vi "Movement sample.vi"() -> ()   [LabVIEW 2018]
uses:
  Underlying VI's/Motor Control VI with PID/MOTOR CONTROL WITH PID AE DIRECTION TYPE DEF.ctl
  Underlying VI's/NavX VI/navX type def.ctl
  Underlying VI's/Motor Control VI with PID/MOTOR CONTROL WITH PID AE DATA MODE TYPE DEF.ctl
  <vilib>/Studica/Studica Toolkit/Background/I2C Channel.ctl
  <vilib>/Studica/Studica Toolkit/NavX/NavX.lvlib
  <vilib>/Studica/Studica Toolkit/Background/DIO Channel.ctl
panel:
  in  "navx mode":T1=enum."Read Values"
  out "NavX Readings":T2
  in  "Speed":dbl
  in  "Direction":T3
  out "Speed & distance 2":T4
  in  "stop":bool
  out "Arduino Data":T5
  out "error out":errorcluster
  in  "Stop program":bool
  out "Mode":T6(ring)
  in  "Boolean":bool
  out "Yaw":dbl
  out "Speed & distance":T4
  in  "error in (no error)":errorcluster
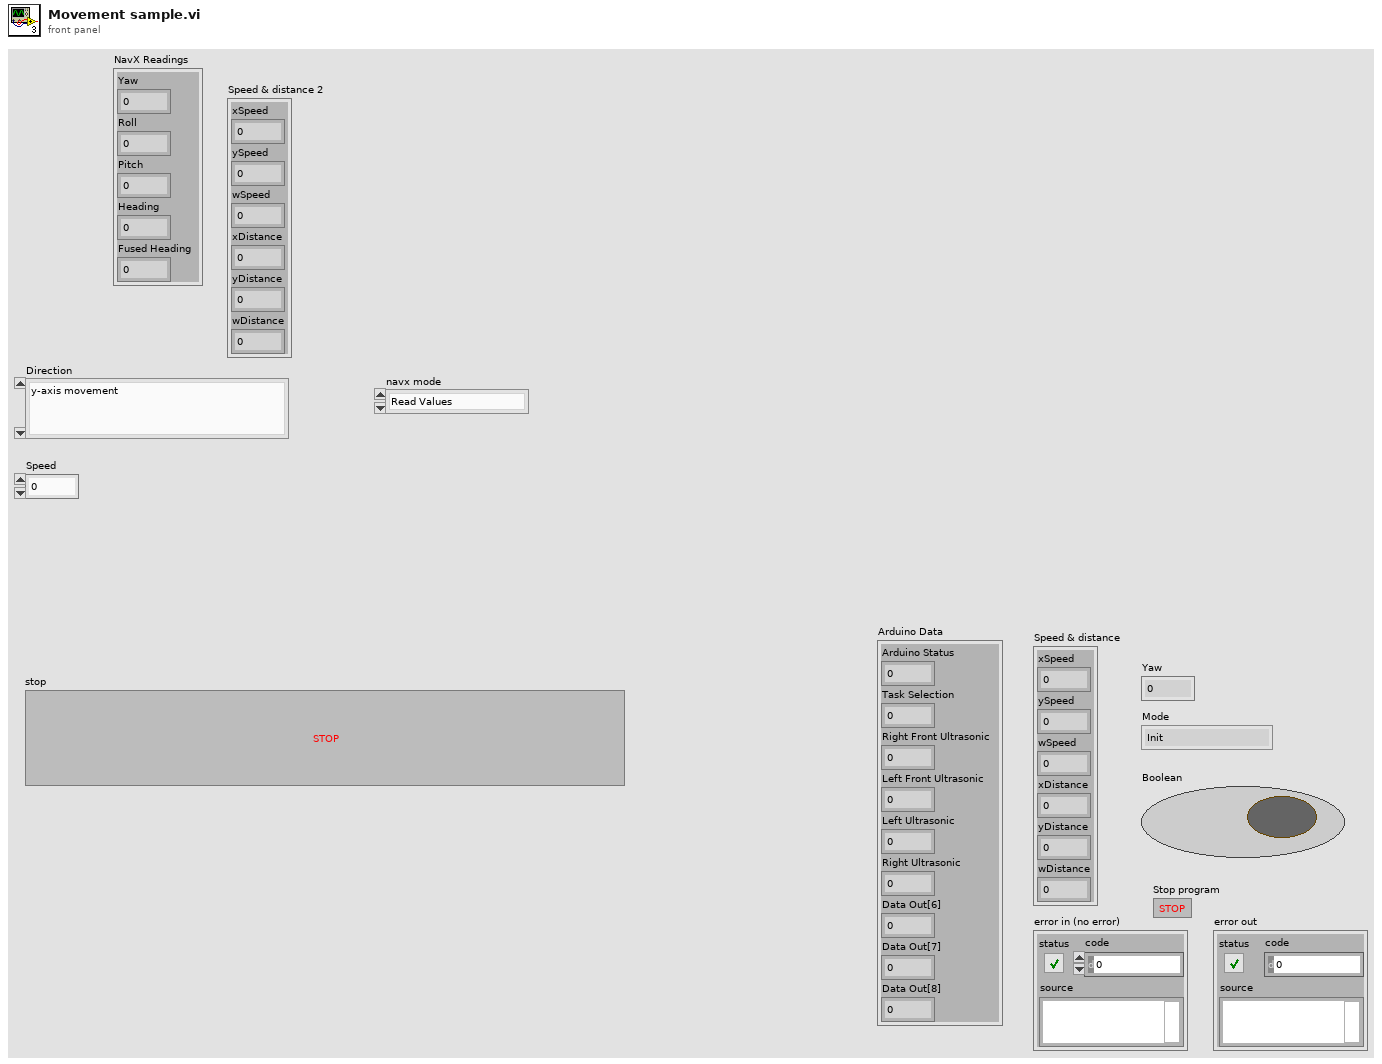
[diagram p1: front panel]
types:
  T1 = typedef "navX type def.ctl" = enum16{"Get i2C reference", "Read Values", "Zero Yaw"}
  T2 = cluster{"Yaw":dbl, "Roll":dbl, "Pitch":dbl, "Heading":dbl, "Fused Heading":dbl}
  T3 = typedef "MOTOR CONTROL WITH PID AE DIRECTION TYPE DEF.ctl" = enum16{"y-axis movement", "x-axis movement", "rotation", "stop", "reset encoders"}
  T4 = cluster{"xSpeed":dbl, "ySpeed":dbl, "wSpeed":dbl, "xDistance":dbl, "yDistance":dbl, "wDistance":dbl}
  T5 = cluster{"Arduino Status":u8, "Task Selection":u8, "Right Front Ultrasonic":u8, "Left Front Ultrasonic":u8, "Left Ultrasonic":u8, "Right Ultrasonic":u8, "Data Out[6]":u8, "Data Out[7]":u8, "Data Out[8]":u8}
  T6 = enum16{"Init", "Front Back", "Left Right", "Rotate", "Latch"}
  T7 = typedef "MOTOR CONTROL WITH PID AE DATA MODE TYPE DEF.ctl" = enum16{"Init AE", "Write to AE", "Read from AE"}
  T8 = typedef "DIO Channel.ctl" = enum16{"Not Connected", "A/DIO1", "A/DIO2", "A/DIO3", "A/DIO4", "A/DIO5", "A/DIO6", "A/DIO7", "A/DIO13", "B/DIO1", "B/DIO2", "B/DIO3", "B/DIO4", "B/DIO5", "B/DIO6", "B/DIO7", "B/DIO13", "C/DIO0", "C/DIO1", "C/DIO2", "C/DIO3", "C/DIO4", "C/DIO5", "C/DIO6", "C/DIO7"}
  T9 = typedef "I2C Channel.ctl" = enum16{"Not Connected", "A", "B"}
  T10 = cluster{"DIO Channel":T8, "FPGA VI Reference Out":refnum<k20>}
  T11 = cluster{"I2C Ref Out":cluster{"I2C Channel":T9, "FPGA VI Reference Out":refnum<k20>}, "Connected":bool, "Slave Address (7-bit)":u8, "Registry":u8[]}
  T12 = cluster{"Arduino Status":u8, "Task Selection":u8, "PING_A":u8, "PING_B":u8, "PING_C":u8, "PING_D":u8, "Compass Low Byte":u8, "Compass High Byte":u8, "Data Out[8]":u8}
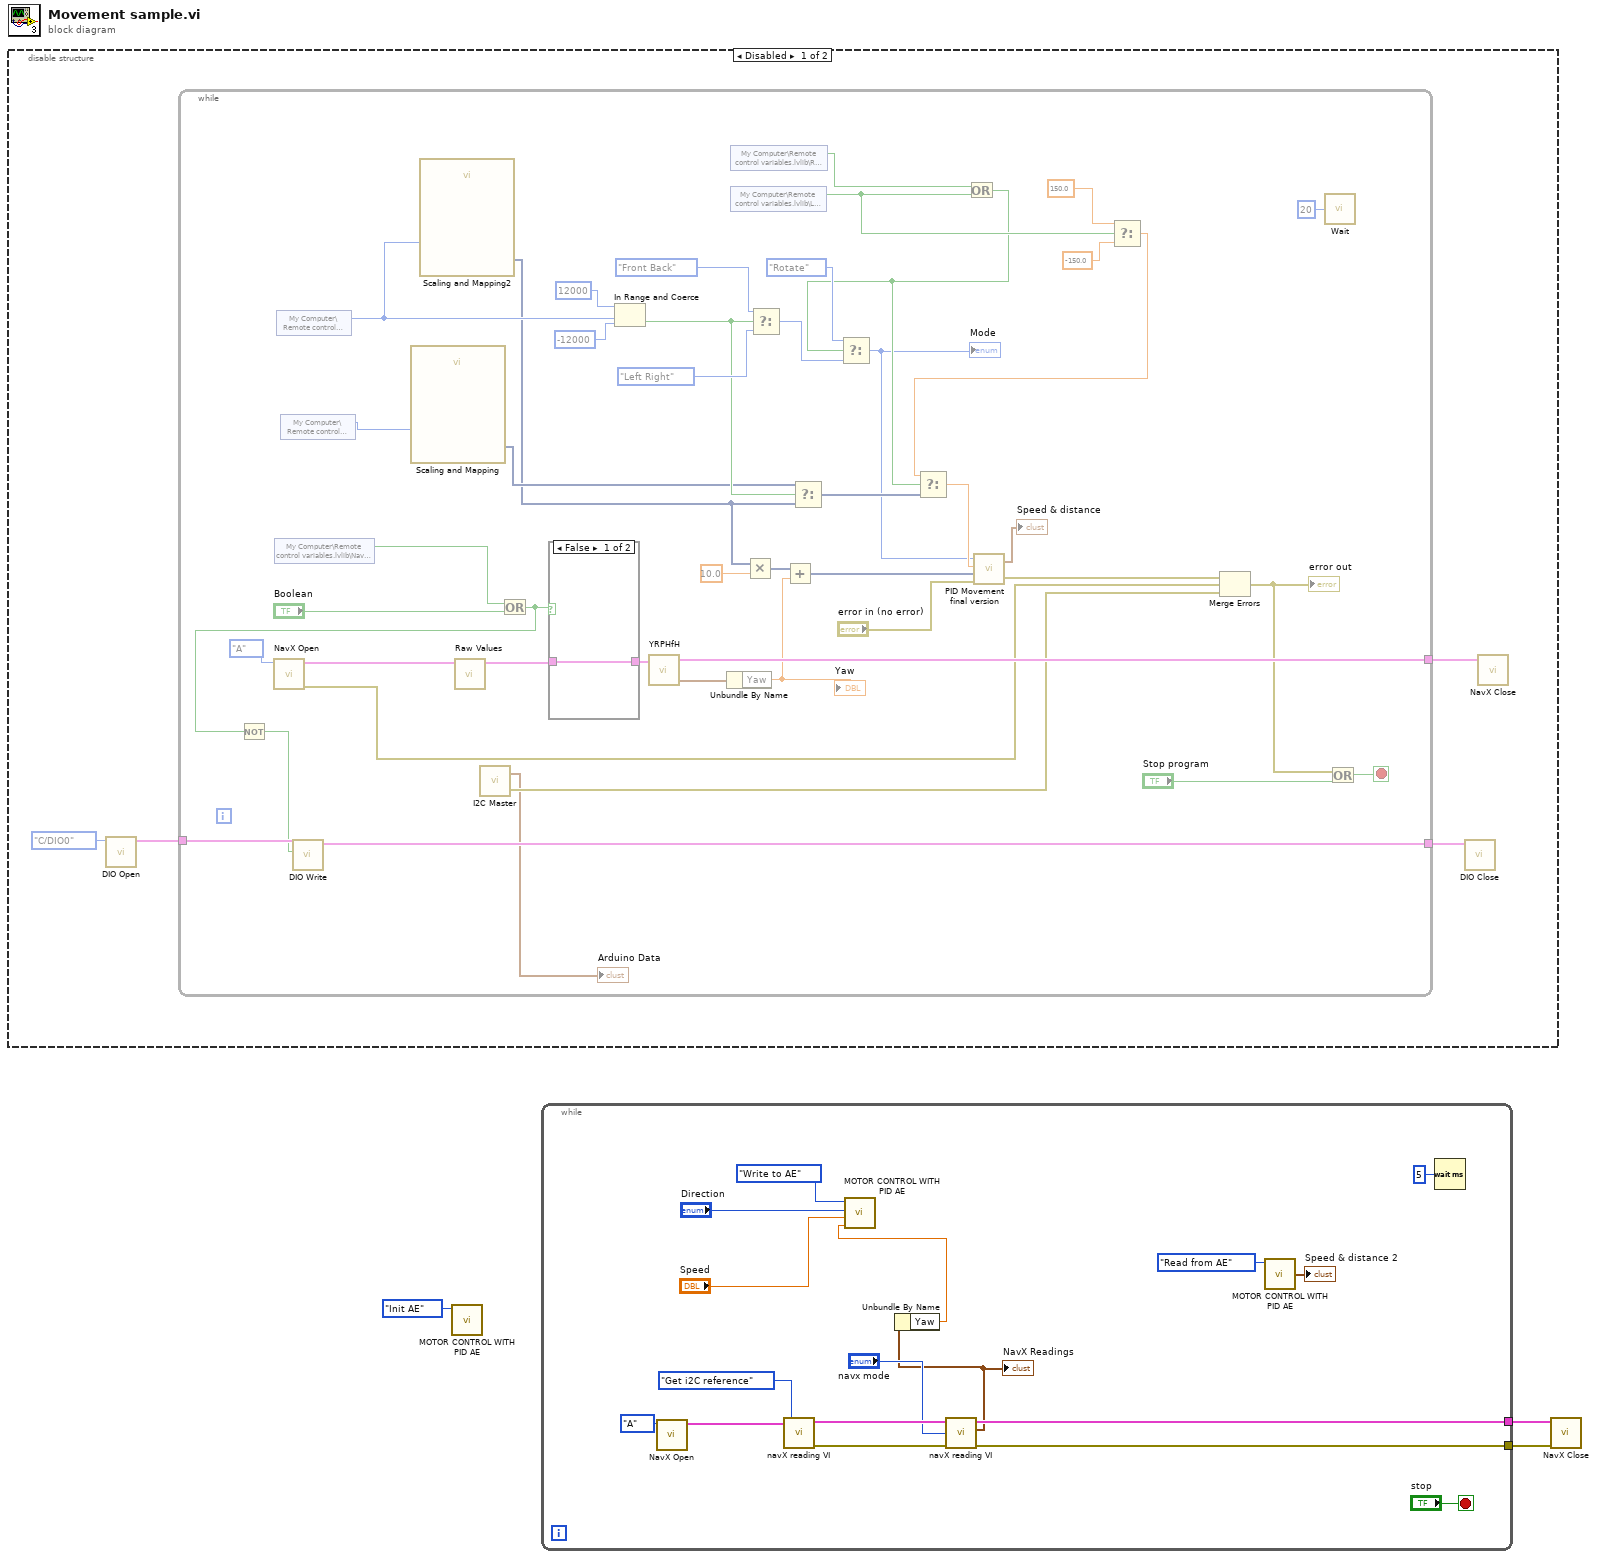
[diagram p0: block diagram]
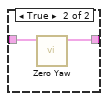
[diagram p2: hidden frame]
diagram:
  n1 = disable-structure shown="Disabled" {
    frame Disabled {
      n2 = call <vilib>:"DIO Open.vi"("DIO Channel"=DIO_Channel."C/DIO0") -> ("DIO Info Out"=w6:T10)  [unwired: 9 in, 1 out]
      n3 = while {
        tunnel: [w49] -> w7
        tunnel: w6 -> [w13]
        tunnel: [w10] -> w4
        stop <- w17 stop-if-true
        n4 = call <vilib>:"NavX Open.vi"("I2C Channel"=I2C_Channel."A") -> ("error out"=w18:errorcluster, "NavX Info"=w47:T11)  [unwired: 9 in]
        n5 = shared-variable "My Computer\\Remote control variables.lvlib\\NavX Stop"() -> (w42:bool)  [unwired: 1 in, 1 out]
        n6 = shared-variable "My Computer\\Remote control variables.lvlib\\X axis"() -> (w41:i32)  [unwired: 1 in, 1 out]
        n7 = shared-variable "My Computer\\Remote control variables.lvlib\\Y axis"() -> (w44:i32)  [unwired: 1 in, 1 out]
        n8 = call "Scaling and Mapping"("Signals"=w44) -> ("Scaled Signals"=w35:dynamicdata)  [unwired: 9 in, 1 out]
        n9 = call "Scaling and Mapping2"("Signals"=w41) -> ("Scaled Signals"=w32:dynamicdata)  [unwired: 9 in, 1 out]
        n10 = call <vilib>:"Raw Values.vi"("NavX Info In"=w47) -> ("NavX Info Out"=w45:T11)  [unwired: 8 in, 1 out]
        n11 = call "I2C Master.vi"() -> ("I2C Error"=w9:errorcluster, "Arduino Data"=→"Arduino Data":T12)  [unwired: 2 in]
        n12 = Or(x=w42, y="Boolean") -> (x .or. y?=w11:bool)
        n13 = Not(x=w11) -> (.not. x?=w12:bool)
        n14 = call <vilib>:"DIO Write.vi"("Input"=w12, "DIO Info In"=w13) -> ("DIO Info Out"=w10:T10)  [unwired: 8 in, 1 out]
        n15 = case shown="False" w11 {
          tunnel: [w54 w56] -> w46
          tunnel: w45 -> [w54 w55]
          frame False {
          }
          frame True {
            n16 = call <vilib>:"Zero Yaw.vi"("NavX Info In"=w55) -> ("NavX Info Out"=w56:T11)  [unwired: 10 in]
          }
        }
        n17 = In Range and Coerce(upper limit=12000, x=w41, lower limit=-12000) -> (In Range?=w36:bool)  [unwired: 1 out]
        n18 = call <vilib>:"YRPHfH.vi"("NavX Info In"=w46) -> ("YRPHfH"=w50:T2, "NavX Info Out"=w49:T11)  [unwired: 3 in]
        n19 = Unbundle By Name(w50) -> ("Yaw"=w20:dbl)
        "Yaw" <- w20
        n20 = shared-variable "My Computer\\Remote control variables.lvlib\\R Bumper"() -> (w30:bool)  [unwired: 1 in, 1 out]
        n21 = shared-variable "My Computer\\Remote control variables.lvlib\\L Bumper"() -> (w27:bool)  [unwired: 1 in, 1 out]
        n22 = Multiply(x=w32, y=10.0) -> (x*y=w33:dynamicdata)
        n23 = Select(t=T6."Front Back" ("Direction"), s=w36, f=T6."Left Right" ("Direction")) -> (s? t:f=w29:T6)
        n24 = Add(x=w33, y=w20) -> (x+y=w34:dynamicdata)
        n25 = Select(t=w35, s=w36, f=w32) -> (s? t:f=w24:dynamicdata)
        n26 = Or(x=w30, y=w27) -> (x .or. y?=w22:bool)
        n27 = Select(t=T6."Rotate", s=w22, f=w29) -> (s? t:f=w14:T6)
        "Mode" <- w14
        n28 = Select(t=150.0, s=w27, f=-150.0) -> (s? t:f=w23:dbl)
        n29 = Select(t=w23, s=w22, f=w24) -> (s? t:f=w21:dbl)
        n30 = call "PID Movement final version.vi"("error in (no error)"="error in (no error)", "Yaw"=w34, "Speed"=w21, "Direction"=w14) -> ("error out"=w19:errorcluster, "Speed & distance"=→"Speed & distance":T4)
        n31 = Merge Errors(w19, w18, w9) -> (w16:errorcluster)
        "error out" <- w16
        n32 = call "Wait"("Count(uSec)"=u32 20) -> ()  [unwired: 1 out]
        n33 = Or(x=w16, y="Stop program") -> (x .or. y?=w17:bool)
      }
      n34 = call <vilib>:"DIO Close.vi"("DIO Info In"=w4) -> ()  [unwired: 10 in, 1 out]
      n35 = call <vilib>:"NavX Close.vi"("NavX Info In"=w7) -> ()  [unwired: 10 in, 1 out]
    }
    frame Enabled {
    }
  }
  n36 = call "MOTOR CONTROL WITH PID AE.vi"("AE Mode"=MOTOR_CONTROL_WITH_PID_AE_DATA_MODE_TYPE_DEF."Init AE") -> ()  [unwired: 3 in, 1 out]
  n37 = while {
    tunnel: [w60] -> w2
    tunnel: [w59] -> w1
    stop <- "stop" stop-if-true
    n38 = call <vilib>:"NavX Open.vi"("I2C Channel"=I2C_Channel."A") -> ("NavX Info"=w65:T11)  [unwired: 9 in, 1 out]
    n39 = call "navX reading VI.vi"("NavX Info In"=w65, "Mode"=navX_type_def."Get i2C reference") -> ("NavX Info Out"=w63:T11, "Error Out"=w62:errorcluster)  [unwired: 1 in, 2 out]
    n40 = call "navX reading VI.vi"("NavX Info In"=w63, "Mode"="navx mode", "error in (no error)"=w62) -> ("NavX Info Out"=w60:T11, "NavX Readings"=w58:T2, "Error Out"=w59:errorcluster)  [unwired: 1 out]
    "NavX Readings" <- w58
    n41 = Unbundle By Name(w58) -> ("Yaw"=w57:dbl)
    n42 = call "MOTOR CONTROL WITH PID AE.vi"("Yaw"=w57, "Speed"="Speed", "Direction"="Direction", "AE Mode"=MOTOR_CONTROL_WITH_PID_AE_DATA_MODE_TYPE_DEF."Write to AE") -> ()  [unwired: 1 out]
    n43 = call "MOTOR CONTROL WITH PID AE.vi"("AE Mode"=MOTOR_CONTROL_WITH_PID_AE_DATA_MODE_TYPE_DEF."Read from AE") -> ("Speed & distance"=→"Speed & distance 2":T4)  [unwired: 3 in]
    n44 = Wait (ms)(milliseconds to wait=u32 5) -> ()  [unwired: 1 out]
  }
  n45 = call <vilib>:"NavX Close.vi"("error in (no error)"=w1, "NavX Info In"=w2) -> ()  [unwired: 9 in, 1 out]
